vi "Auton Playback.vi"(0 "copilot fifo":refnum<k33>, 1 "driver fifo":refnum<k33>, 2 "Copilot FName":string, 3 "Driver FName":string) -> ()   [LabVIEW 2014]
uses:
  TeleopCmd.ctl
  CmdFlag.ctl
  Co-Pilot_game_control.ctl
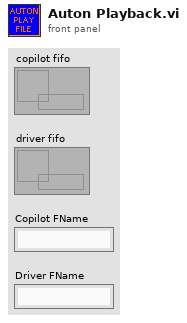
[diagram p1: front panel]
types:
  T1 = typedef "Co-Pilot_game_control.ctl" = cluster{"Left_Intake":dbl, "Right_Intake":dbl, "Time Stamp":u32, "Command":enum16{"Noop", "Flagged"}, "ToggleCollector":bool, "ManualLift":dbl, "Top_Limit_Switch":bool, "Bottom_Limit_Switch ":bool, "LifterOverride":bool, "AutoLift":i32, "Toggle Auto Lifter":bool, "Activate HP indexer":bool}
  T2 = typedef "TeleopCmd.ctl" = cluster{"CmdFlag":T3, "throttle":dbl, "turn":dbl, "Override":bool, "Strafe":dbl, "MotorPwrMax":u8, "Time":u32, "ultrasonic override":bool}
  T3 = typedef "CmdFlag.ctl" = enum16{"noop", "logflag", "suspend", "resume"}
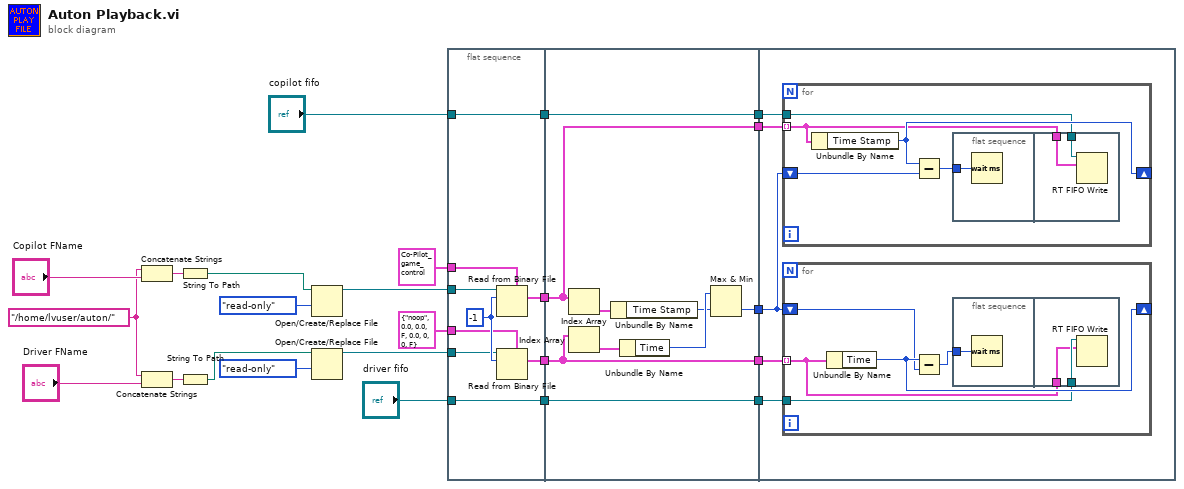
[diagram p0: block diagram]
diagram:
  w1 = "/home/lvuser/auton/" ("string")
  n1 = Concatenate Strings(w1, "Copilot FName") -> (w4:string)
  n2 = Concatenate Strings(w1, "Driver FName") -> (w2:string)
  n3 = String To Path(string=w4) -> (path=w24:path)
  n4 = String To Path(string=w2) -> (path=w21:path)
  n5 = Open/Create/Replace File(file path (use dialog)=w24, access (0:read/write)=enum16{"read/write", "read-only", "write-only"}."read-only") -> (refnum out=w16:refnum<file>)  [unwired: 4 in, 2 out]
  n6 = Open/Create/Replace File(file path (use dialog)=w21, access (0:read/write)=enum16{"read/write", "read-only", "write-only"}."read-only") -> (refnum out=w15:refnum<file>)  [unwired: 4 in, 2 out]
  n7 = flat-sequence {
    tunnel: "driver fifo" -> [w33]
    tunnel: [w33] -> w14
    tunnel: T2 {"CmdFlag"=enum."noop", "throttle"=0.0, "turn"=0.0, "Override"=FALSE, "Strafe"=0.0, "MotorPwrMax"=0, "Time"=0, "ultrasonic override"=FALSE} ("Cluster") -> [w31]
    tunnel: T1 {"Left_Intake"=0.0, "Right_Intake"=0.0, "Time Stamp"=0, "Command"=enum."Noop", "ToggleCollector"=FALSE, "ManualLift"=0.0, "Top_Limit_Switch"=FALSE, "Bottom_Limit_Switch "=FALSE, "LifterOverride"=FALSE, "AutoLift"=0, "Toggle Auto Lifter"=FALSE, "Activate HP indexer"=FALSE} -> [w30]
    tunnel: [w29] -> w12
    tunnel: "copilot fifo" -> [w29]
    tunnel: w16 -> [w28]
    tunnel: w15 -> [w27]
    tunnel: [w26] -> w10
    tunnel: [w25] -> w8
    tunnel: w14 -> [w42]
    tunnel: [w42] -> w13
    tunnel: w12 -> [w41]
    tunnel: [w41] -> w11
    tunnel: w10 -> [w39]
    tunnel: [w39] -> w9
    tunnel: w8 -> [w40]
    tunnel: [w40] -> w7
    tunnel: [w34] -> w6
    tunnel: w13 -> [w47]
    tunnel: w11 -> [w46]
    tunnel: w9 -> [w45]
    tunnel: w7 -> [w44]
    tunnel: w6 -> [w43]
    frame #0 {
      w32 = -1 ("count (1)")
      n8 = Read from Binary File(5:w30, 10:w32, 11:w28) -> (2:w25:T1[])  [unwired: 3 in, 3 out]
      n9 = Read from Binary File(5:w31, 10:w32, 11:w27) -> (2:w26:T2[])  [unwired: 3 in, 3 out]
    }
    frame #1 {
      n10 = Index Array(array=w40) -> (element=w38:T1)  [unwired: 1 in]
      n11 = Index Array(array=w39) -> (element=w37:T2)  [unwired: 1 in]
      n12 = Unbundle By Name(w38) -> ("Time Stamp"=w35:u32)
      n13 = Unbundle By Name(w37) -> ("Time"=w36:u32)
      n14 = Max & Min(x=w36, y=w35) -> (min(x,y)=w34:u32)  [unwired: 1 out]
    }
    frame #2 {
      n15 = for {
        tunnel: w46 -> [w49]
        tunnel: w44 -> [w48] mode=indexing
        shift-right: [w51] -> _
        shift-left: w43 -> [w50]
        n16 = Unbundle By Name(w48) -> ("Time Stamp"=w51:u32)
        n17 = Subtract(x=w51, y=w50) -> (x-y=w52:u32)
        n18 = flat-sequence {
          tunnel: w52 -> [w53]
          tunnel: w49 -> [w55]
          tunnel: w48 -> [w54]
          frame #0 {
            n19 = Wait (ms)(milliseconds to wait=w53) -> ()  [unwired: 1 out]
          }
          frame #1 {
            n20 = RT FIFO Write(0:w55, 1:w54) -> ()  [unwired: 3 in, 4 out]
          }
        }
      }
      n21 = for {
        tunnel: w47 -> [w57]
        tunnel: w45 -> [w56] mode=indexing
        shift-right: [w60] -> _
        shift-left: w43 -> [w59]
        n22 = Unbundle By Name(w56) -> ("Time"=w60:u32)
        n23 = Subtract(x=w60, y=w59) -> (x-y=w58:u32)
        n24 = flat-sequence {
          tunnel: w58 -> [w61]
          tunnel: w57 -> [w63]
          tunnel: w56 -> [w62]
          frame #0 {
            n25 = Wait (ms)(milliseconds to wait=w61) -> ()  [unwired: 1 out]
          }
          frame #1 {
            n26 = RT FIFO Write(0:w63, 1:w62) -> ()  [unwired: 3 in, 4 out]
          }
        }
      }
    }
  }
